vi "launch tortoisegit log.vi"() -> ()   [LabVIEW 2018]
uses:
  <vilib>/Utility/error.llb/Error Cluster From Error Code.vi
  <vilib>/ErrorRing/Error Ring.xnode
panel:
  out "return code":i32
  out "standard error":string
  out "standard output 2":string
  out "standard output":string
  out "VI Path":path
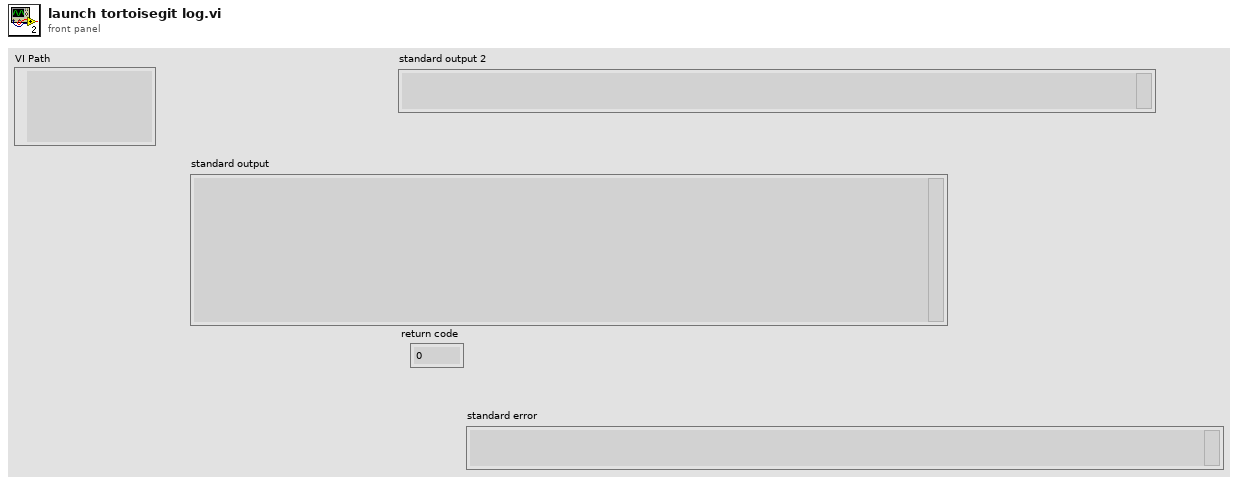
[diagram p1: front panel]
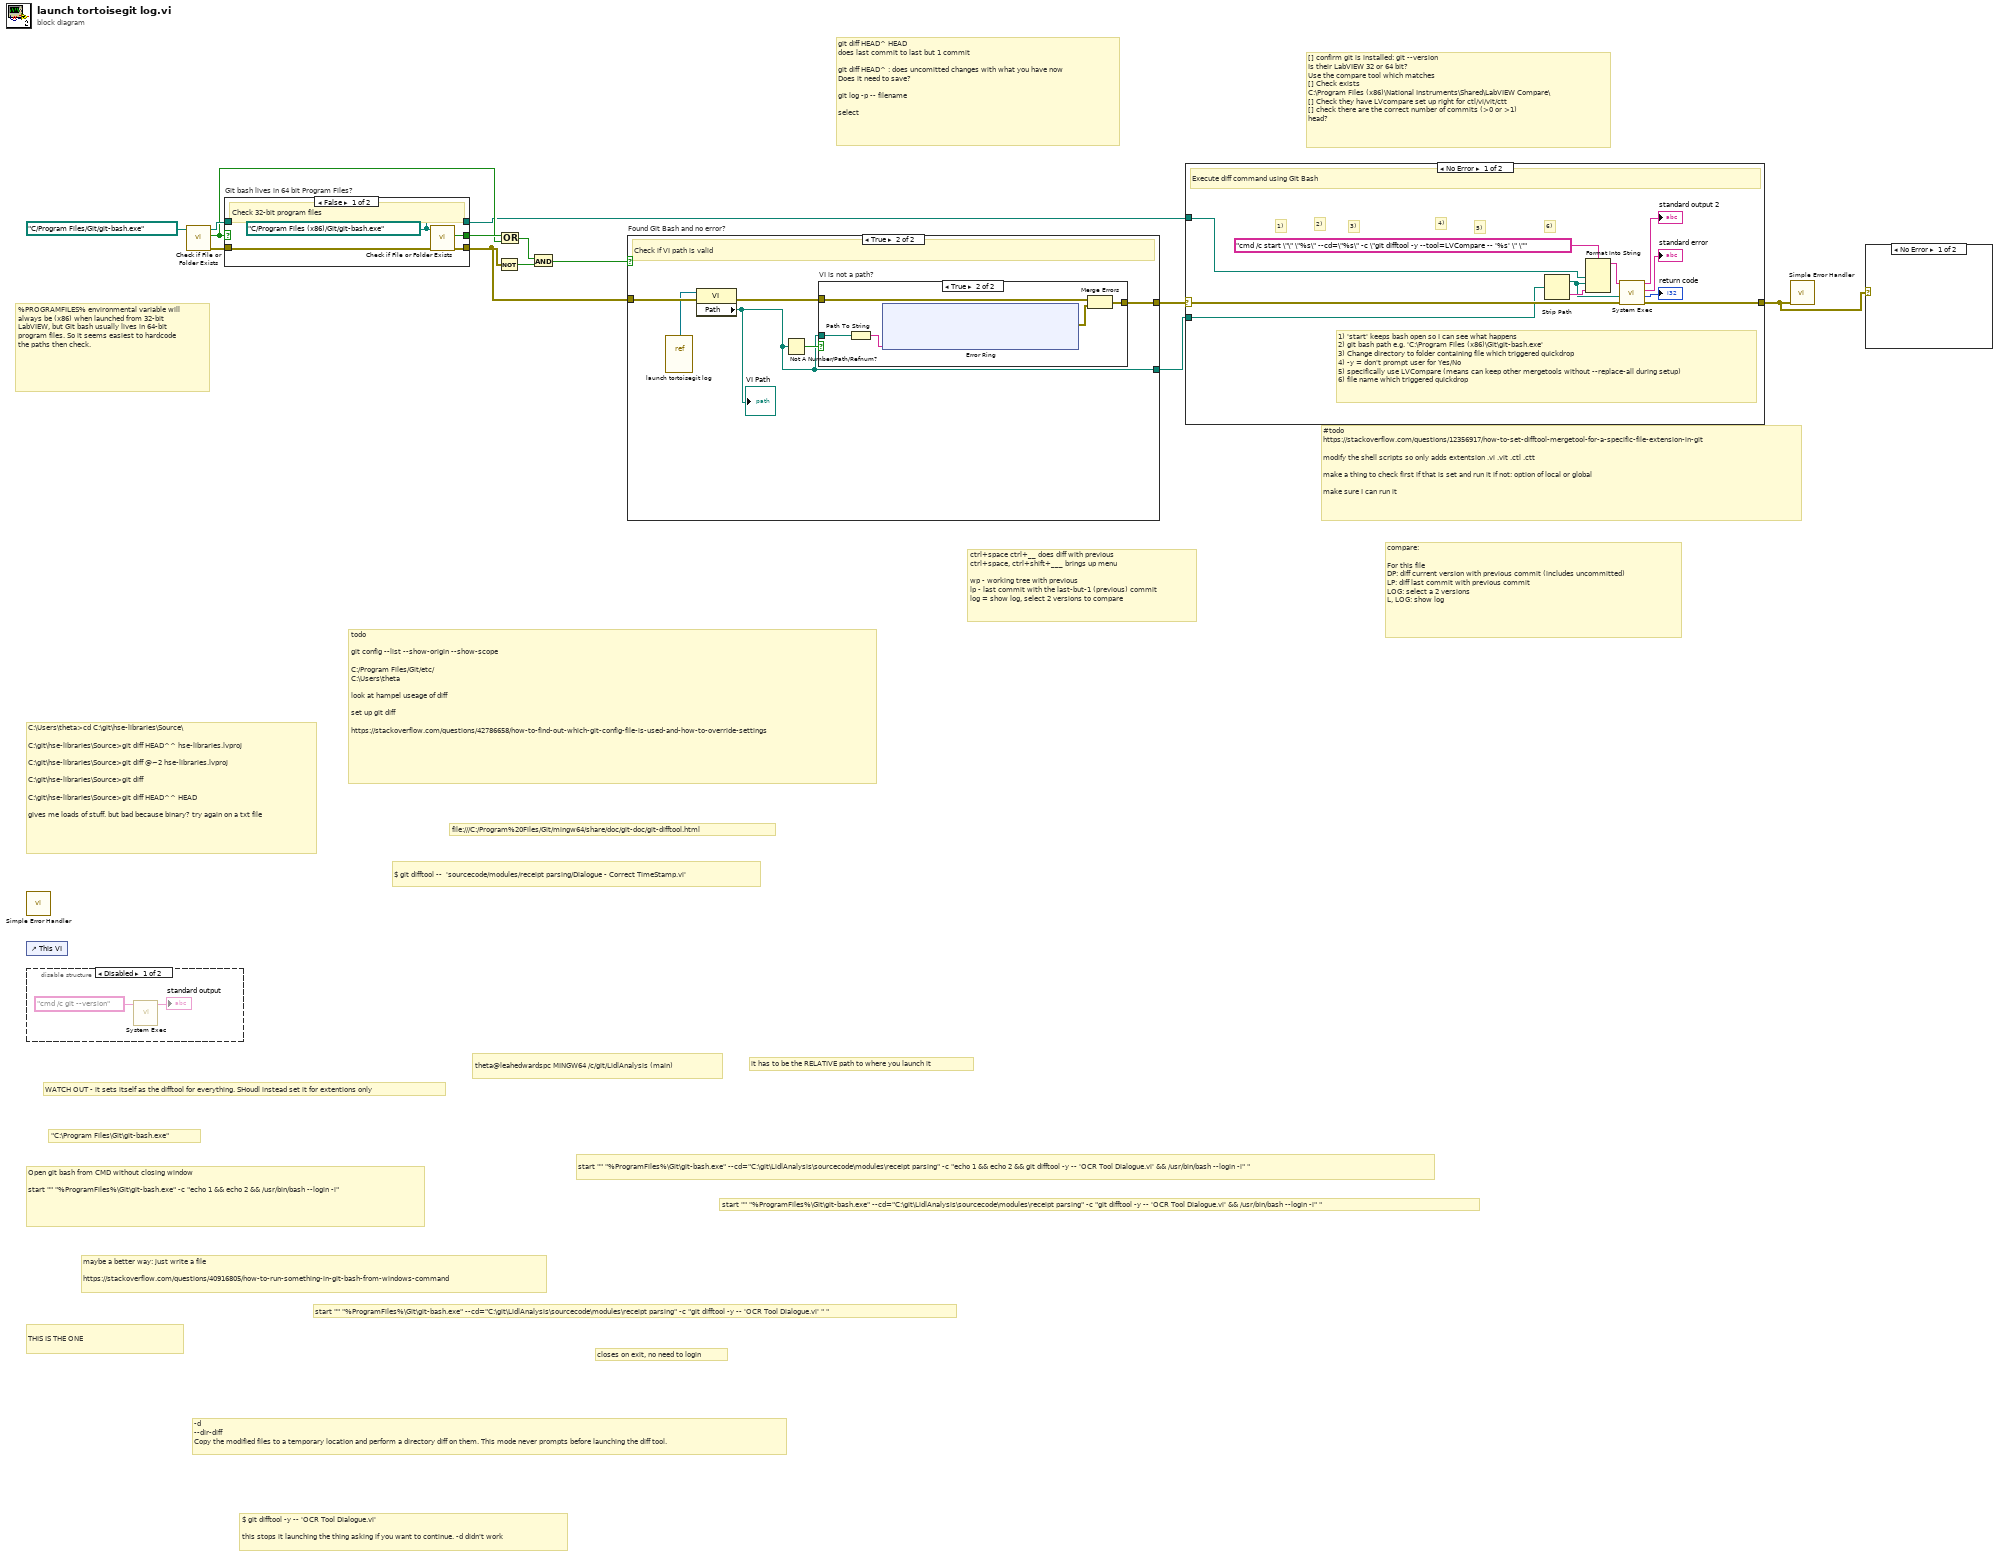
[diagram p0: block diagram]
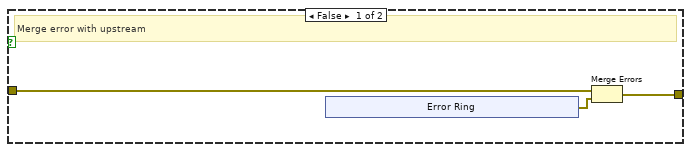
[diagram p4: hidden frame]
diagram:
  # "ctrl+space ctrl+__ does diff with previous\nctrl+space, ctrl+shift+___ brings up menu\n\nwp - working tree with previous\nlp - last commit with the last-but-1 (previous) commit\nlog = show log, select 2 versions to compare"
  # "#todo\nhttps://stackoverflow.com/questions/12356917/how-to-set-difftool-mergetool-for-a-specific-file-extension-in-git\n\nmodify the shell scripts so only adds extentsion .vi .vit .ctl .ctt\n\nmake a thing to check first if that is set and run it if not: option of local or global\n\nmake sure I can run it"
  # "compare:\n\nFor this file\nDP: diff current version with previous commit (includes uncommitted)\nLP: diff last commit with previous commit\nLOG: select a 2 versions\nL, LOG: show log"
  # "%PROGRAMFILES% environmental variable will always be (x86) when launched from 32-bit LabVIEW, but Git bash usually lives in 64-bit program files. So it seems easiest to hardcode the paths then check."
  # "\"C:\\Program Files\\Git\\git-bash.exe\""
  # "closes on exit, no need to login"
  # "$ git difftool -y -- 'OCR Tool Dialogue.vi'\n\nthis stops it launching the thing asking if you want to continue. -d didn't work"
  # "-d\n--dir-diff\nCopy the modified files to a temporary location and perform a directory diff on them. This mode never prompts before launching the diff tool."
  # "THIS IS THE ONE"
  # "start \"\" \"%ProgramFiles%\\Git\\git-bash.exe\" --cd=\"C:\\git\\LidlAnalysis\\sourcecode\\modules\\receipt parsing\" -c \"git difftool -y -- 'OCR Tool Dialogue.vi' \" \""
  # "start \"\" \"%ProgramFiles%\\Git\\git-bash.exe\" --cd=\"C:\\git\\LidlAnalysis\\sourcecode\\modules\\receipt parsing\" -c \"git difftool -y -- 'OCR Tool Dialogue.vi' && /usr/bin/bash --login -i\" \""
  # "start \"\" \"%ProgramFiles%\\Git\\git-bash.exe\" --cd=\"C:\\git\\LidlAnalysis\\sourcecode\\modules\\receipt parsing\" -c \"echo 1 && echo 2 && git difftool -y -- 'OCR Tool Dialogue.vi' && /usr/bin/bash --login -i\" \""
  # "maybe a better way: just write a file\n\nhttps://stackoverflow.com/questions/40916805/how-to-run-something-in-git-bash-from-windows-command"
  # "Open git bash from CMD without closing window\n\nstart \"\" \"%ProgramFiles%\\Git\\git-bash.exe\" -c \"echo 1 && echo 2 && /usr/bin/bash --login -i\""
  # "WATCH OUT - it sets itself as the difftool for everything. SHoudl instead set it for extentions only"
  # "it has to be the RELATIVE path to where you launch it"
  # "theta@leahedwardspc MINGW64 /c/git/LidlAnalysis (main)"
  # "$ git difftool --  'sourcecode/modules/receipt parsing/Dialogue - Correct TimeStamp.vi'"
  # "file:///C:/Program%20Files/Git/mingw64/share/doc/git-doc/git-difftool.html"
  # "C:\\Users\\theta>cd C:\\git\\hse-libraries\\Source\\\n\nC:\\git\\hse-libraries\\Source>git diff HEAD^^ hse-libraries.lvproj\n\nC:\\git\\hse-libraries\\Source>git diff @~2 hse-libraries.lvproj\n\nC:\\git\\hse-libraries\\Source>git diff\n\nC:\\git\\hse-libraries\\Source>git diff HEAD^^ HEAD\n\ngives me loads of stuff. but bad because binary? try again on a txt file"
  # "todo\n\ngit config --list --show-origin --show-scope\n\nC:/Program Files/Git/etc/\nC:\\Users\\theta\n\nlook at hampel useage of diff\n\nset up git diff\n\nhttps://stackoverflow.com/questions/42786658/how-to-find-out-which-git-config-file-is-used-and-how-to-override-settings"
  # "[] confirm git is installed: git --version\nIs their LabVIEW 32 or 64 bit?\nUse the compare tool which matches\n[] Check exists\nC:\\Program Files (x86)\\National Instruments\\Shared\\LabVIEW Compare\\\n[] Check they have LVcompare set up right for ctl/vi/vit/ctt\n[] check there are the correct number of commits (>0 or >1)\nhead?"
  # "git diff HEAD^ HEAD\ndoes last commit to last but 1 commit\n\ngit diff HEAD^ : does uncomitted changes with what you have now\nDoes it need to save?\n\ngit log -p -- filename\n\nselect"
  n1 = call <vilib>:"Simple Error Handler.vi"() -> ()  [unwired: 5 in, 5 out]
  n2 = control-ref of="This VI"() -> ()  [unwired: 1 out]
  n3 = disable-structure shown="Disabled" {
    frame Disabled {
      n4 = call <vilib>:"System Exec.vi"("command line"="cmd /c git --version") -> ("standard output"=→"standard output":string)  [unwired: 7 in, 3 out]
    }
    frame Enabled {
    }
  }
  n5 = call <vilib>:"Check if File or Folder Exists.vi"("path"=path "C:/Program Files/Git/git-bash.exe") -> ("error out"=w11:errorcluster, "file or folder exists?"=w9:bool, "dup path"=w12:path)  [unwired: 8 in]
  n6 = case "Git bash lives in 64 bit Program Files?" shown="False" w9 {
    tunnel: w12 -> [_ w21]
    tunnel: w11 -> [w19 w20]
    tunnel: [w18 _] -> w10
    tunnel: [w17 w21] -> w4
    tunnel: [w16 w20] -> w6
    frame False {
      w17 = path "C:/Program Files (x86)/Git/git-bash.exe" ("path")
      # "Check 32-bit program files"
      n7 = call <vilib>:"Check if File or Folder Exists.vi"("error in (no error)"=w19, "path"=w17) -> ("error out"=w16:errorcluster, "file or folder exists?"=w18:bool)  [unwired: 7 in, 1 out]
    }
    frame True {
    }
  }
  n8 = Not(x=w6) -> (.not. x?=w7:bool)
  n9 = Or(x=w10, y=w9) -> (x .or. y?=w8:bool)
  n10 = And(x=w8, y=w7) -> (x .and. y?=w5:bool)
  n11 = case "Found Git Bash and no error?" shown="True" w5 {
    tunnel: w6 -> [w24 w35]
    tunnel: [w22 w33] -> w3
    tunnel: [_ w31] -> w2
    frame False {
      # "Merge error with upstream"
      n12 = xnode "Error Ring"() -> ("error out"=w23:errorcluster)
      n13 = Merge Errors(w24, w23) -> (w22:errorcluster)
    }
    frame True {
      # "Check if VI path is valid"
      n14 = vi-ref "launch tortoisegit log.vi"() -> (w30:refnum<vi>)
      n15 = property class="VI"(reference=w30, error in=w35) -> (error out=w34:errorcluster, "Path"=w31:path)  [unwired: 1 out]
      "VI Path" <- w31
      n16 = Not A Number/Path/Refnum?(number/path/refnum=w31) -> (NaN/Path/Refnum?=w32:bool)
      n17 = case "VI is not a path?" shown="True" w32 {
        tunnel: w31 -> [_ w41]
        tunnel: w34 -> [w36 w40]
        tunnel: [w36 w38] -> w33
        frame False {
        }
        frame True {
          n18 = Path To String(path=w41) -> (string=w37:string)
          n19 = xnode "Error Ring"("parameter 0"=w37) -> ("error out"=w39:errorcluster)
          n20 = Merge Errors(w40, w39) -> (w38:errorcluster)
        }
      }
    }
  }
  n21 = case shown="No Error" w3 {
    selector: w3 -> [w50 w60]
    tunnel: w4 -> [w52 _]
    tunnel: [w51 w60] -> w1
    tunnel: w2 -> [w49 _]
    frame No Error {
      # "6)"
      # "5)"
      # "1) 'start' keeps bash open so I can see what happens\n2) git bash path e.g. 'C:\\Program Files (x86)\\Git\\git-bash.exe'\n3) Change directory to folder containing file which triggered quickdrop\n4) -y = don't prompt user for Yes/No\n5) specifically use LVCompare (means can keep other mergetools without --replace-all during setup)\n6) file name which triggered quickdrop"
      # "4)"
      # "3)"
      # "2)"
      # "1)"
      # "Execute diff command using Git Bash"
      n22 = Strip Path(path=w49) -> (stripped path=w58:path, name=w59:string)
      n23 = Format Into String(format string="cmd /c start \"\" \"%s\" --cd=\"%s\" -c \"git difftool -y --tool=LVCompare -- '%s' \" \"", w52, w58, w59) -> (resulting string=w54:string)  [unwired: 2 in, 1 out]
      n24 = call <vilib>:"System Exec.vi"("error in (no error)"=w50, "working directory"=w58, "command line"=w54) -> ("error out"=w51:errorcluster, "return code"=→"return code":i32, "standard error"=→"standard error":string, "standard output"=→"standard output 2":string)  [unwired: 5 in]
    }
    frame Error {
    }
  }
  n25 = call <vilib>:"Simple Error Handler.vi"("error in (no error)"=w1) -> ()  [unwired: 4 in, 5 out]
  n26 = case shown="No Error" w1 {
    frame No Error {
    }
    frame Error {
    }
  }
